vi "GetMFCSetPoint.vi"(1 "MFC ID Number":i32) -> (0 "SetPoint":dbl)   [LabVIEW 2011]
uses:
  GlobalVariables.vi
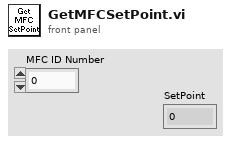
[diagram p1: front panel]
types:
  T1 = typedef "MFC Cluster.ctl" = cluster{"ID Number":u8, "Status":bool[], "Flow (SCCM)":dbl, "SetPoint (SCCM)":dbl, "Actuator Override":i8, "Actuator Drive Valve":i16, "Setpoint Output":dbl}
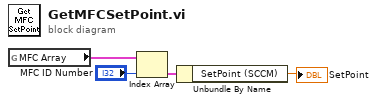
[diagram p0: block diagram]
diagram:
  n1 = global read "GlobalVariables.vi" "MFC Array"() -> (w4:T1[])
  n2 = Index Array(array=w4, index="MFC ID Number") -> (element=w2:T1)
  n3 = Unbundle By Name(w2) -> ("SetPoint (SCCM)"=→"SetPoint":dbl)
